vi "Reset All Shift Data.vi"(11 "refnum in":T1) -> (3 "refnum out":T1)   [LabVIEW 2018]
uses:
  <vilib>/Utility/config.llb/Config Data RefNum.ctl
  <vilib>/Utility/config.llb/NI_LVConfig.lvlib
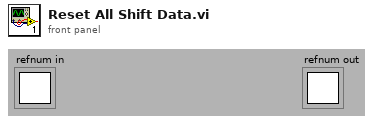
[diagram p1: front panel]
types:
  T1 = typedef "NI_LVConfig.lvlib/Config Data RefNum.ctl" = refnum<k1>
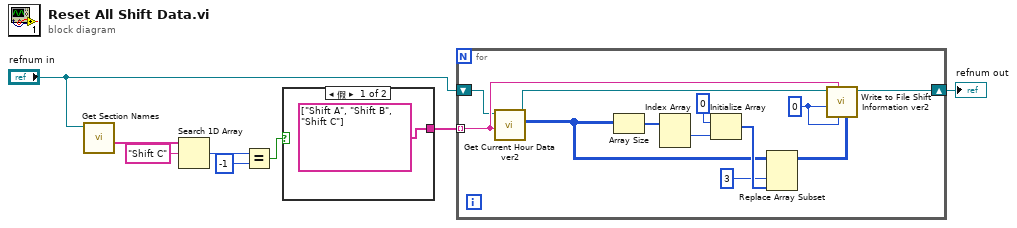
[diagram p0: block diagram]
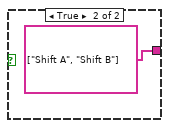
[diagram p2: hidden frame]
diagram:
  n1 = call <vilib>:"Get Section Names.vi"("refnum"="refnum in") -> ("section names"=w6:string[])  [unwired: 8 in, 2 out]
  n2 = Search 1D Array(1D array=w6, element="Shift C") -> (index of element=w4:i32)  [unwired: 1 in]
  n3 = Equal?(x=w4, y=-1) -> (x = y?=w1:bool)
  n4 = case shown="假" w1 {
    tunnel: [string[] ["Shift A", "Shift B", "Shift C"] string[] ["Shift A", "Shift B"]] -> w8
    frame False {
    }
    frame True {
    }
  }
  n5 = for {
    tunnel: w8 -> [w15] mode=indexing
    shift-right: [w13] -> w7
    shift-left: "refnum in" -> [w12]
    w22 = u32 0 ("Actual Per Shift")
    n6 = call "Get Current Hour Data ver2.vi"("Shift"=w15, "Refnum in"=w12) -> ("Shift Hour Data"=w16:u32[][], "Refnum Out"=w14:T1)  [unwired: 5 in, 3 out]
    n7 = Array Size(array=w16) -> (size(s)=w18:i32[])
    n8 = Index Array(array=w18) -> (element #1=w11:i32)  [unwired: 2 in, 1 out]
    n9 = Initialize Array(u32 0 ("Current Hour Actual"), w11) -> (w21:u32[])
    n10 = Replace Array Subset(array=w16, new element=w21, index (col)=3 ("disabled index (col)")) -> (w17:u32[][])  [unwired: 1 in]
    n11 = call "Write to File Shift Information ver2.vi"("Shift Hour Data"=w17, "Reject"=w22, "Shift"=w15, "Actual Per Shift"=w22, "Refnum in"=w14) -> ("refnum out"=w13:T1)  [unwired: 5 in, 1 out]
  }
  "refnum out" <- w7
